vi "Test Helper Loop Cannot Launch Outside Process.vi"(8 "error in (no error)":errorcluster, 11 "Helper Loop Test In":refnum<class "Helper Loop Test.lvclass">) -> (0 "error out":errorcluster, 3 "Helper Loop Test Out":refnum<class "Helper Loop Test.lvclass">)   [LabVIEW 2020, in "Helper Loop Test.lvclass"]
uses:
  Helper Loop Test.lvclass
  C:/Program Files (x86)/National Instruments/LabVIEW 2020/vi.lib/Astemes/LUnit/Test Case.lvclass
  source/Framework Test Suite/Mock Process/Mock Process.lvclass
  C:/Git/astemes-triarc-framework/source/Framework/Process/Process.lvclass
  <vilib>/Astemes/LUnit/Test Case.lvclass/Test Case.ctl
  <vilib>/Astemes/LUnit/LUnit Assertion Result.lvclass/LUnit Assertion Result.ctl
  <vilib>/Astemes/LUnit/LUnit Test Case Result.lvclass/LUnit Test Case Result.ctl
  <vilib>/Astemes/LUnit/LUnit Method Result.lvclass/LUnit Method Result.ctl
  source/Framework/Process/Process.lvclass/Process.ctl
  <vilib>/Astemes/LUnit/Palette/Fail.vi
  <vilib>/Astemes/LUnit/Palette/Pass.vi
  <vilib>/Astemes/LUnit/Set Assertion Type.vi
  source/Framework/Process/Private/SubVIs/Wait for finish.vi
  source/Framework/Process/Protected/Messaging/Enqueue Message.vi
  source/Framework/Process/Private/SubVIs/Set Lifecycle State.vi
  source/Framework/Process/Public/Lifecycle/Get Lifecycle State.vi
  <vilib>/Astemes/LUnit/Add test result.vi
  <vilib>/Astemes/LUnit/LUnit Write Passed.vi
  <vilib>/Astemes/LUnit/LUnit Write Message.vi
  <vilib>/Astemes/LUnit/LUnit Write Description.vi
  <vilib>/Astemes/LUnit/LUnit Write Assertion Type.vi
  source/Framework/Process/Private/SubVIs/Handle Debug Data.vi
  <vilib>/Utility/error.llb/Clear Errors.vi
  <vilib>/Astemes/LUnit/LUnit Record Assertion Result.vi
  source/Framework/Logging/Log Debug.vi
  <vilib>/AdvancedString/1D String Array to Delimited String.vi
  <vilib>/Utility/High Resolution Relative Seconds.vi
  <vilib>/Astemes/LUnit/LUnit Aggregate Assertion Results.vi
  <vilib>/Astemes/LUnit/Assertion Result/LUnit Read Status.vi
  <vilib>/Astemes/LUnit/LUnit Read Message.vi
  <vilib>/Astemes/LUnit/LUnit Read Description.vi
  <vilib>/Astemes/LUnit/Method Result/LUnit Merge Status.vi
  <vilib>/Astemes/LUnit/LUnit Concatenate result strings.vi
  <vilib>/Utility/error.llb/Error Cluster From Error Code.vi
  source/Framework/Process/Public/Read Name.vi
  <vilib>/Astemes/LUnit/LUnit Assertion Result.lvclass
  source/Framework/Process/Process.lvclass
  Helper Loop Test.lvclass/Helper Loop Test.ctl
  <vilib>/Astemes/LUnit/Test Case.lvclass
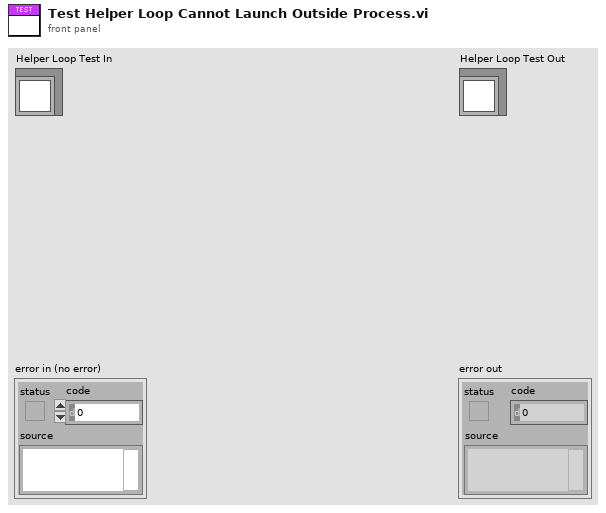
[diagram p1: front panel]
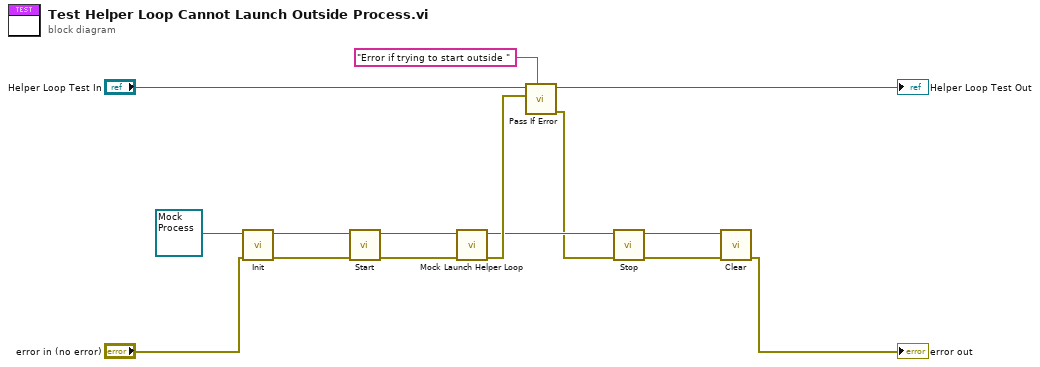
[diagram p0: block diagram]
diagram:
  n1 = call-dynamic "Init.vi"("error in (no error)"="error in (no error)", "Mock Process In"=refnum<class "Mock Process.lvclass"> refnum ("Mock Process.lvclass")) -> ("error out"=w8:errorcluster, "Mock Process Out"=w13:refnum<class "Mock Process.lvclass">)  [unwired: 8 in]
  n2 = call "Start.vi"("error in (no error)"=w8, "Process In"=w13) -> ("error out"=w7:errorcluster, "Process Out"=w12:refnum<class "Mock Process.lvclass">)  [unwired: 7 in, 1 out]
  n3 = call "Mock Launch Helper Loop.vi"("error in (no error)"=w7, "Mock Process in"=w12) -> ("error out"=w10:errorcluster, "Mock Process out"=w9:refnum<class "Mock Process.lvclass">)  [unwired: 8 in]
  n4 = call <vilib>:"Pass If Error.vi"("Description"="Error if trying to start outside ", "Assert error"=w10, "LUnit Test Case In"="Helper Loop Test In") -> ("error out"=w4:errorcluster, "LUnit Test Case Out"=→"Helper Loop Test Out":refnum<class "Helper Loop Test.lvclass">)  [unwired: 7 in]
  n5 = call "Stop.vi"("error in (no error)"=w4, "Process In"=w9) -> ("error out"=w5:errorcluster, "Process Out"=w6:refnum<class "Mock Process.lvclass">)  [unwired: 7 in, 1 out]
  n6 = call-dynamic "Clear.vi"("error in (no error)"=w5, "Mock Process In"=w6) -> ("error out"=→"error out":errorcluster)  [unwired: 9 in]
